vi "Handle Parameter Configuration File Change.vi"(8 "error in":errorcluster, 10 "new parameter configuration file path":path, 11 "custom device ref":T1 format="%.0x") -> (0 "error out":errorcluster, 2 "parameters configuration file out":path, 3 "custom device ref out":T1 format="%.0x")   [LabVIEW 2020, in "AIM MIL-STD-1553 System Explorer.lvlib" / "Implementation.lvlib" / "Refresh.lvlib"]
uses:
  Refresh.lvlib
  Scripting/AIM MIL-STD-1553 Scripting.lvlib
  Import/MIL-STD 1553 Import.lvlib
  Implementation.lvlib
  Shared/Address.ctl
  Shared/Major Frame Definition.ctl
  Shared/Minor Frame Definition.ctl
  Shared/Message Type.ctl
  Shared/Terminal Endpoint.ctl
  Shared/Parameter Definition.ctl
  Shared/Message Definition.ctl
  Shared/BIU Configuration.ctl
  <vilib>/NI VeriStand/Custom Device API/Custom Device Item Ref.ctl
  <vilib>/NI VeriStand/Custom Device API/Custom Device API.lvlib
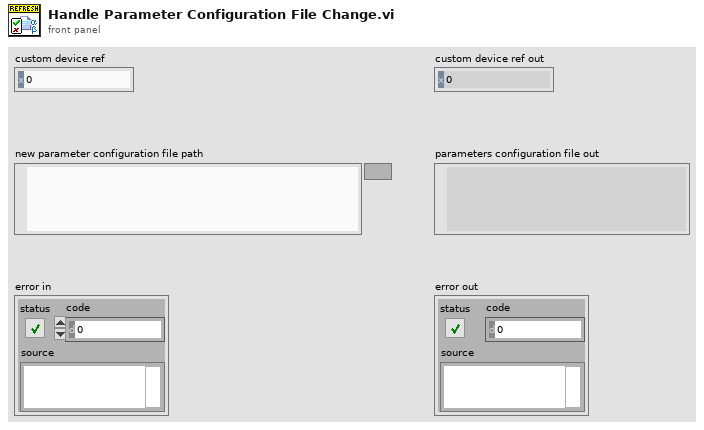
[diagram p1: front panel]
types:
  T1 = typedef "Custom Device API.lvlib/Custom Device Item Ref.ctl" = u64
  T2 = typedef "BIU Configuration.ctl" = cluster{"HW channel":u16, "terminal addresses":T3[], "terminal names":string[], "acyclic frame names":string[], "major frames":T4[], "minor frames":T5[], "messages":T6[]}
  T3 = typedef "Address.ctl" = u16
  T4 = typedef "Major Frame Definition.ctl" = cluster{"name":string, "minor frames":string[]}
  T5 = typedef "Minor Frame Definition.ctl" = cluster{"name":string, "messages":string[]}
  T6 = typedef "Message Definition.ctl" = cluster{"name":string, "message type":T7, "endpoint Tx":T8, "endpoint Rx":T8, "create timestamp channel":bool, "mode code":u16, "number of words":u16, "parameters":cluster{"name":string, "default value":dbl, "unit":string, "parameter definition":T9}[]}
  T7 = typedef "Message Type.ctl" = string
  T8 = typedef "Terminal Endpoint.ctl" = cluster{"terminal address":T3, "subaddress":T3}
  T9 = typedef "Parameter Definition.ctl" = cluster{"start index":i32, "size (bits)":i32, "encoding":enum16{"BNR", "BCD", "Discrete"}, "signed":bool, "multiplier":dbl, "offset":dbl}
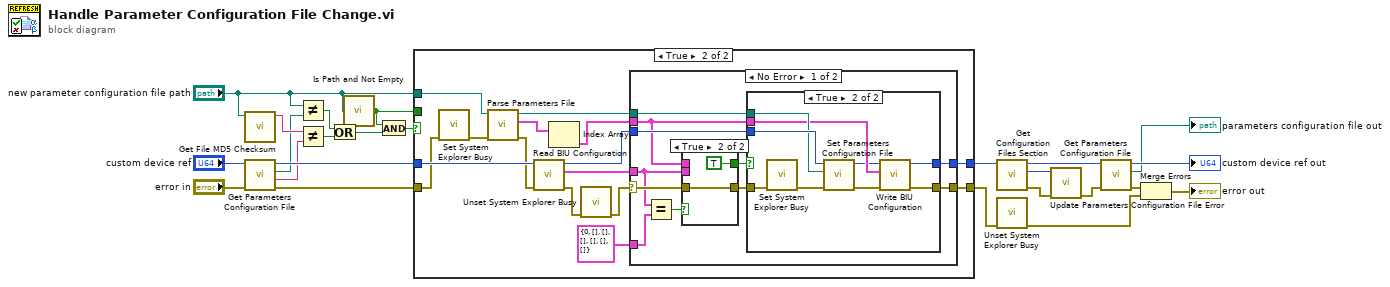
[diagram p0: block diagram]
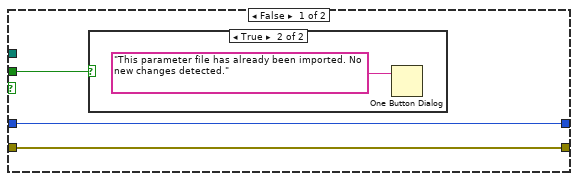
[diagram p2: hidden frame]
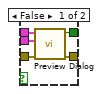
[diagram p4: hidden frame]
diagram:
  n1 = call "Get File MD5 Checksum.vi"("path"="new parameter configuration file path") -> ("MD5"=w17:string)  [unwired: 9 in, 1 out]
  n2 = call "Get Parameters Configuration File.vi"("error in"="error in", "custom device"="custom device ref") -> ("error out"=w24:errorcluster, "MD5 checksum"=w20:string, "parameters configuration file"=w4:path, "custom device out"=w22:T1)  [unwired: 6 in]
  n3 = Not Equal?(x="new parameter configuration file path", y=w4) -> (x != y?=w19:bool)
  n4 = Not Equal?(x=w17, y=w20) -> (x != y?=w18:bool)
  n5 = Or(x=w19, y=w18) -> (x .or. y?=w16:bool)
  n6 = call <vilib>:"Is Path and Not Empty.vi"("path"="new parameter configuration file path") -> ("Is Path and Not Empty?"=w14:bool)  [unwired: 4 in]
  n7 = And(x=w14, y=w16) -> (x .and. y?=w15:bool)
  n8 = case shown="True" w15 {
    tunnel: w24 -> [w25 w34]
    tunnel: w22 -> [w26 w42]
    tunnel: "new parameter configuration file path" -> [_ w43]
    tunnel: w14 -> [w27 _]
    tunnel: [w26 w41] -> w9
    tunnel: [w25 w40] -> w2
    frame False {
      n9 = case shown="True" w27 {
        frame False {
        }
        frame True {
          n10 = One Button Dialog(message="This parameter file has already been imported. No new changes detected.") -> ()  [unwired: 1 in, 1 out]
        }
      }
    }
    frame True {
      n11 = call "Set System Explorer Busy.vi"("error in"=w34) -> ("error out"=w33:errorcluster)  [unwired: 10 in]
      n12 = call "Parse Parameters File.vi"("error in"=w33, "path to XML document"=w43) -> ("error out"=w39:errorcluster, "biu configuration"=w31:T2[], "path to XML document out"=w36:path)  [unwired: 7 in]
      n13 = call "Read BIU Configuration.vi"("error in"=w39, "custom device"=w42) -> ("error out"=w35:errorcluster, "biu configuration"=w38:T2, "custom device out"=w37:T1)  [unwired: 7 in]
      n14 = Index Array(array=w31) -> (element=w30:T2)  [unwired: 1 in]
      n15 = call "Unset System Explorer Busy.vi"("error in"=w35) -> ("error out"=w32:errorcluster)  [unwired: 10 in]
      n16 = case shown="No Error" w32 {
        selector: w32 -> [w54 w73]
        tunnel: w30 -> [w47 _]
        tunnel: w38 -> [w45 _]
        tunnel: [w49 w74] -> w41
        tunnel: w37 -> [w51 w74]
        tunnel: [w48 w73] -> w40
        tunnel: w36 -> [w50 _]
        tunnel: T2 {"HW channel"=0, "terminal addresses"=[], "terminal names"=[], "acyclic frame names"=[], "major frames"=[], "minor frames"=[], "messages"=[]} ("biu configuration") -> [w46 _]
        frame No Error {
          n17 = Equal?(x=w45, y=w46) -> (x = y?=w44:bool)
          n18 = case shown="True" w44 {
            tunnel: w54 -> [w59 w60]
            tunnel: [w58 TRUE ("apply changes")] -> w53
            tunnel: [w57 w60] -> w52
            tunnel: w47 -> [w56 _]
            tunnel: w45 -> [w55 _]
            frame False {
              n19 = call "Preview Dialog.vi"("error in"=w59, "current configuration"=w55, "new configuration"=w56) -> ("error out"=w57:errorcluster, "apply changes"=w58:bool)  [unwired: 7 in]
            }
            frame True {
            }
          }
          n20 = case shown="True" w53 {
            tunnel: w52 -> [w62 w66]
            tunnel: w51 -> [w63 w72]
            tunnel: w50 -> [_ w71]
            tunnel: w47 -> [_ w70]
            tunnel: [w63 w69] -> w49
            tunnel: [w62 w68] -> w48
            frame False {
            }
            frame True {
              n21 = call "Set System Explorer Busy.vi"("error in"=w66) -> ("error out"=w67:errorcluster)  [unwired: 10 in]
              n22 = call "Set Parameters Configuration File.vi"("error in"=w67, "parameters configuration file path"=w71, "custom device"=w72) -> ("error out"=w64:errorcluster, "custom device out"=w65:T1)  [unwired: 7 in]
              n23 = call "Write BIU Configuration.vi"("error in"=w64, "biu configuration"=w70, "custom device"=w65) -> ("error out"=w68:errorcluster, "custom device out"=w69:T1)  [unwired: 7 in]
            }
          }
        }
        frame Error {
        }
      }
    }
  }
  n24 = call "Get Configuration Files Section.vi"("custom device"=w9) -> ("error out"=w10:errorcluster, "configuration files section"=w11:T1, "custom device out"=w13:T1)  [unwired: 7 in, 1 out]
  n25 = call "Unset System Explorer Busy.vi"("error in"=w2) -> ("error out"=w1:errorcluster)  [unwired: 10 in]
  n26 = call "Update Parameters Configuration File Error.vi"("error in"=w10, "configuration files section"=w11) -> ("error out"=w12:errorcluster)  [unwired: 8 in, 1 out]
  n27 = call "Get Parameters Configuration File.vi"("error in"=w12, "custom device"=w13) -> ("error out"=w8:errorcluster, "parameters configuration file"=→"parameters configuration file out":path, "custom device out"=→"custom device ref out":T1)  [unwired: 6 in, 1 out]
  n28 = Merge Errors(w8, w1) -> (→"error out":errorcluster)
